vi "Goalie Normal.vi"(9 "balls":T1[](array[typedef]), 10 "Robot in":T3, 11 "IA State":T2={"our_robots"=[], "enemy_robots"=[], "balls"=[], "geometry"={"field_length"=0, "field_width"=0, "goal_width"=0, "goal_depth"=0, "center_circle_radius"=0, "defense_width"=0, "defense_depth"=0, "free_kick_from_defense_dist"=0, "penalty_spot_from_field_line_dist"=0, "penalty_line_from_spot_dist"=0, "half_moon_depth"=0, "half_moon_width"=0}, "IA Judge"={"stage"="", "command"="", "our_goalie_id"=0.0, "enemy_goalie_id"=0.0, "command enum"=enum."Halt", "Time"=enum."Azul"}, "Received Timestamp"=timestamp(0 s since 1904-01-01), "Events"={"Touch"=FALSE, "id touch"=0.0, "Ball out of \nVision"=FALSE, "Ball inside \nGoalie area"=FALSE, "Robot not responding"=FALSE, "Robots responding status"=[1.0, 1.0, 1.0, 1.0, 1.0, 1.0], "Enemy Ball \nPossession"=FALSE, "Id ini Possession"=0.0, "Ball Possesion"=FALSE, "Id Possesion"=0.0, "Ball at\nour goal side"=FALSE, "Ball at\ntouchline"=FALSE, "Ball at\nenemy goal side"=FALSE}}) -> (3 "Robot out":T3)   [LabVIEW 2017]
uses:
  Core/AI Robot.ctl
  Functions Enum.ctl
  AttackerStates.ctl
  Path Planning/RRT/PathDests.ctl
  Path Planning/RRT/PathDest.ctl
  Core/AI Input.ctl
  Core/AI Ball.ctl
  Core/Field Size.ctl
  Core/AI Judge.ctl
  Command Enum.ctl
  Util/Events/Events.ctl
  <vilib>/Analysis/_algsub.llb/Real Vector Norm.vi
  <vilib>/Analysis/NI_AALPro.lvlib
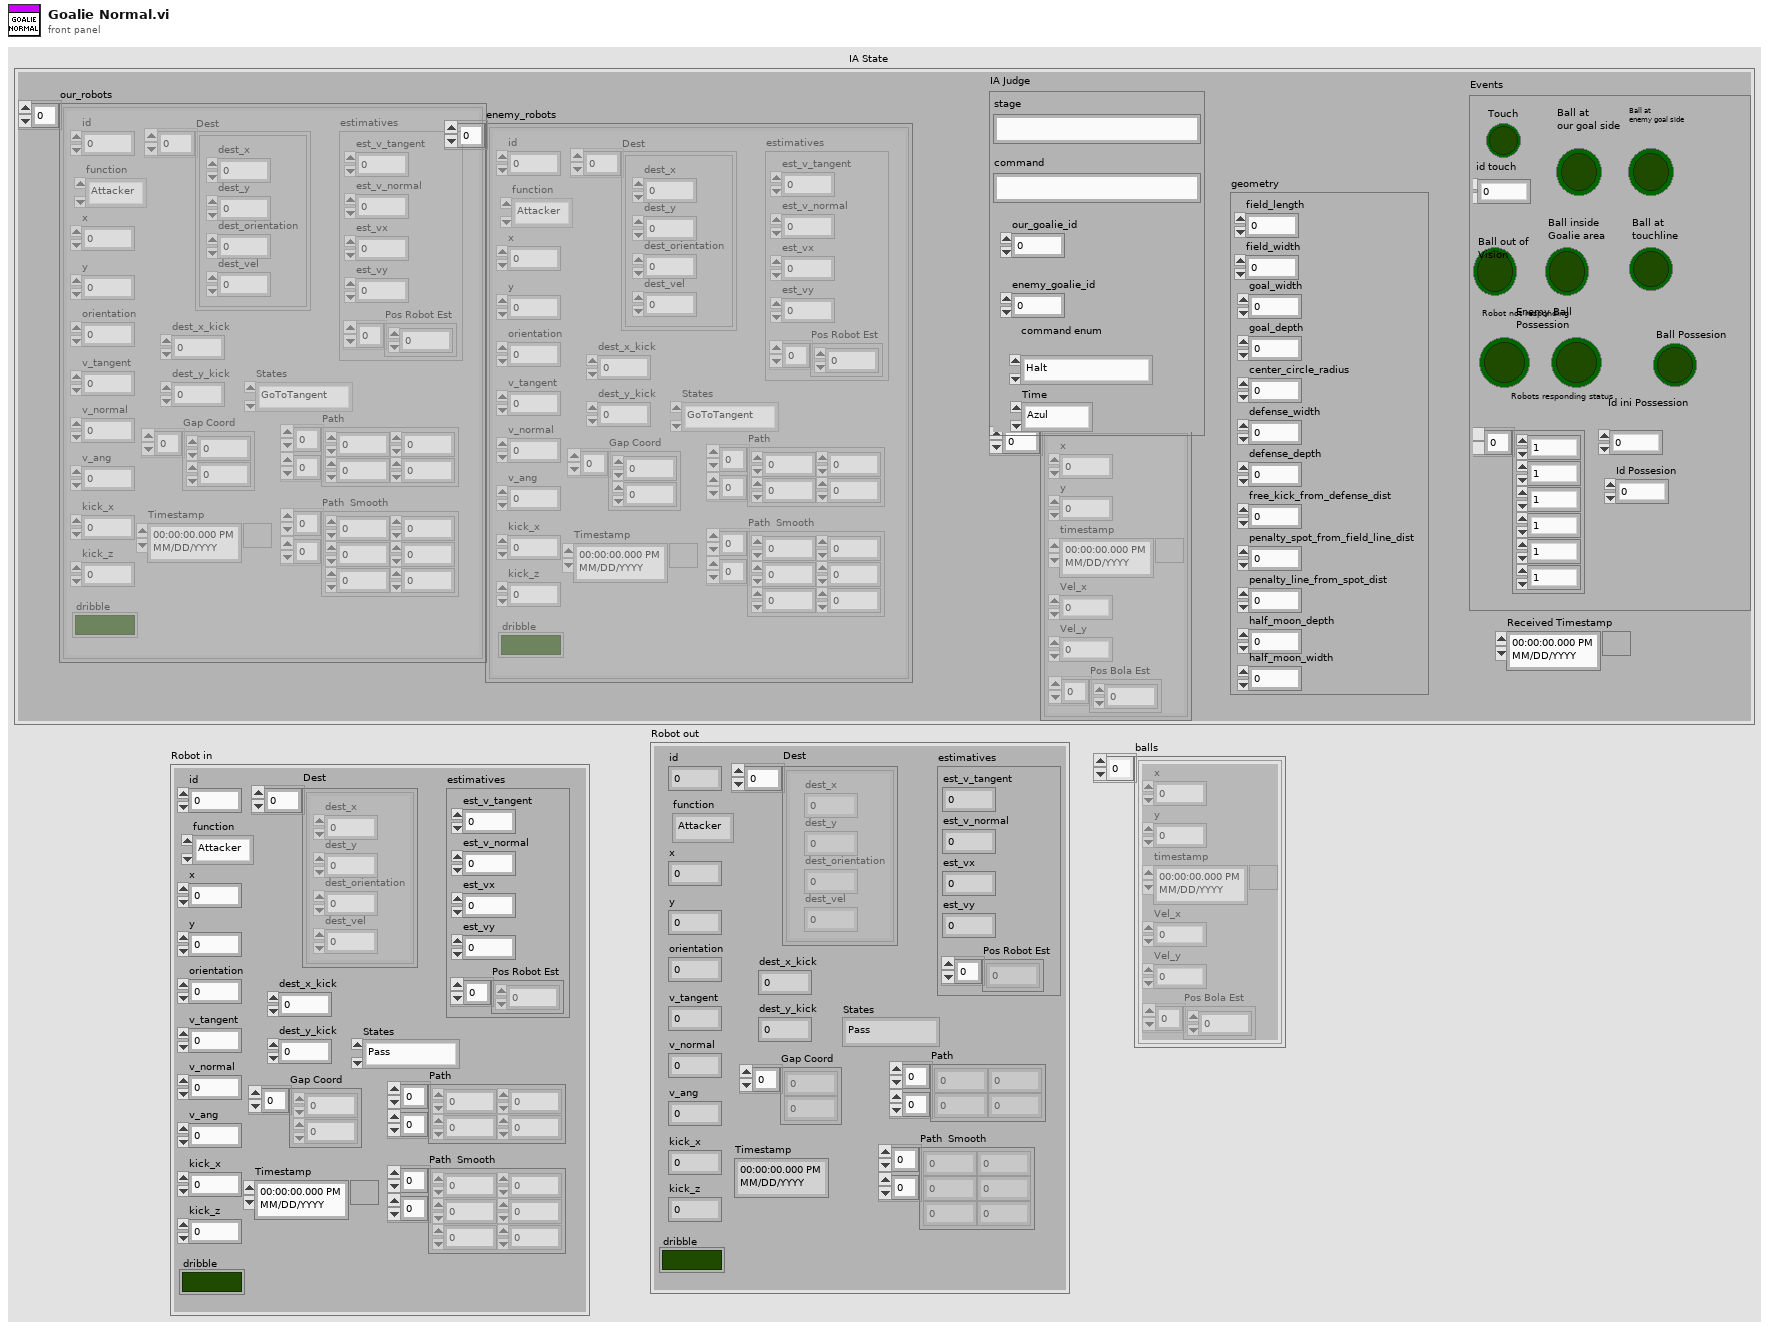
[diagram p1: front panel]
types:
  T1 = typedef "AI Ball.ctl" = cluster{"x":dbl, "y":dbl, "timestamp":timestamp, "Vel_x":dbl, "Vel_y":dbl, "Pos Bola Est":dbl[]}
  T2 = typedef "AI Input.ctl" = cluster{"our_robots":T3[], "enemy_robots":T3[], "balls":T1[], "geometry":T8, "IA Judge":T9, "Received Timestamp":timestamp, "Events":T11}
  T3 = typedef "AI Robot.ctl" = cluster{"id":u32, "function":T4, "x":dbl, "y":dbl, "orientation":dbl, "v_tangent":dbl, "v_normal":dbl, "v_ang":dbl, "kick_x":dbl, "kick_z":dbl, "dribble":bool, "Timestamp":timestamp, "estimatives":cluster{"est_v_tangent":dbl, "est_v_normal":dbl, "est_vx":dbl, "est_vy":dbl, "Pos Robot Est":dbl[]}, "dest_x_kick":dbl, "dest_y_kick":dbl, "Gap Coord":dbl[], "States":T5, "Path ":dbl[][], "Path  Smooth":dbl[][], "Dest":T6}
  T4 = typedef "Functions Enum.ctl" = enum16{"Attacker", "Goalie", "Defender", "Striker", "Goto 0", "Dummy", "Kicker", "ZigZag"}
  T5 = typedef "AttackerStates.ctl" = enum16{"Pass", "GoToTangent", "BallGetting", "GoToKick", "Rotate anti-clockwise", "Rotate Clockwise", ""}
  T6 = typedef "PathDests.ctl" = T7[]
  T7 = typedef "PathDest.ctl" = cluster{"dest_x":dbl, "dest_y":dbl, "dest_orientation":dbl, "dest_vel":dbl}
  T8 = typedef "Field Size.ctl" = cluster{"field_length":u32, "field_width":u32, "goal_width":u32, "goal_depth":u32, "center_circle_radius":u32, "defense_width":u32, "defense_depth":u32, "free_kick_from_defense_dist":u32, "penalty_spot_from_field_line_dist":u32, "penalty_line_from_spot_dist":u32, "half_moon_depth":u32, "half_moon_width":u32}
  T9 = typedef "AI Judge.ctl" = cluster{"stage":string, "command":string, "our_goalie_id":dbl, "enemy_goalie_id":dbl, "command enum":T10, "Time":enum16{"Azul", "Amarelo"}}
  T10 = typedef "Command Enum.ctl" = enum16{"Halt", "Stop", "Force Start", "PKA Normal Start", "Prepare Kickoff Ally", "PKE Normal Start", "Prepare Kickoff Enemy", "Prepare Penalty Ally", "PPA Normal Start", "Prepare Penalty Enemy", "PPE Normal Start", "Direct Free Enemy", "Direct Free Ally", "Indirect Free Enemy", "Indirect Free Ally", "Timeout Enemy", "Timeout Ally", "Goal Enemy", "Goal Ally", "Ball Placement Enemy", "Ball Placement Ally", "Normal Half Time", "Extra Time Break", "Extra Half Time", "None", "Post Game"}
  T11 = typedef "Events.ctl" = cluster{"Touch":bool, "id touch":dbl, "Ball out of \nVision":bool, "Ball inside \nGoalie area":bool, "Robot not responding":bool, "Robots responding status":dbl[], "Enemy Ball \nPossession":bool, "Id ini Possession":dbl, "Ball Possesion":bool, "Id Possesion":dbl, "Ball at\nour goal side":bool, "Ball at\ntouchline":bool, "Ball at\nenemy goal side":bool}
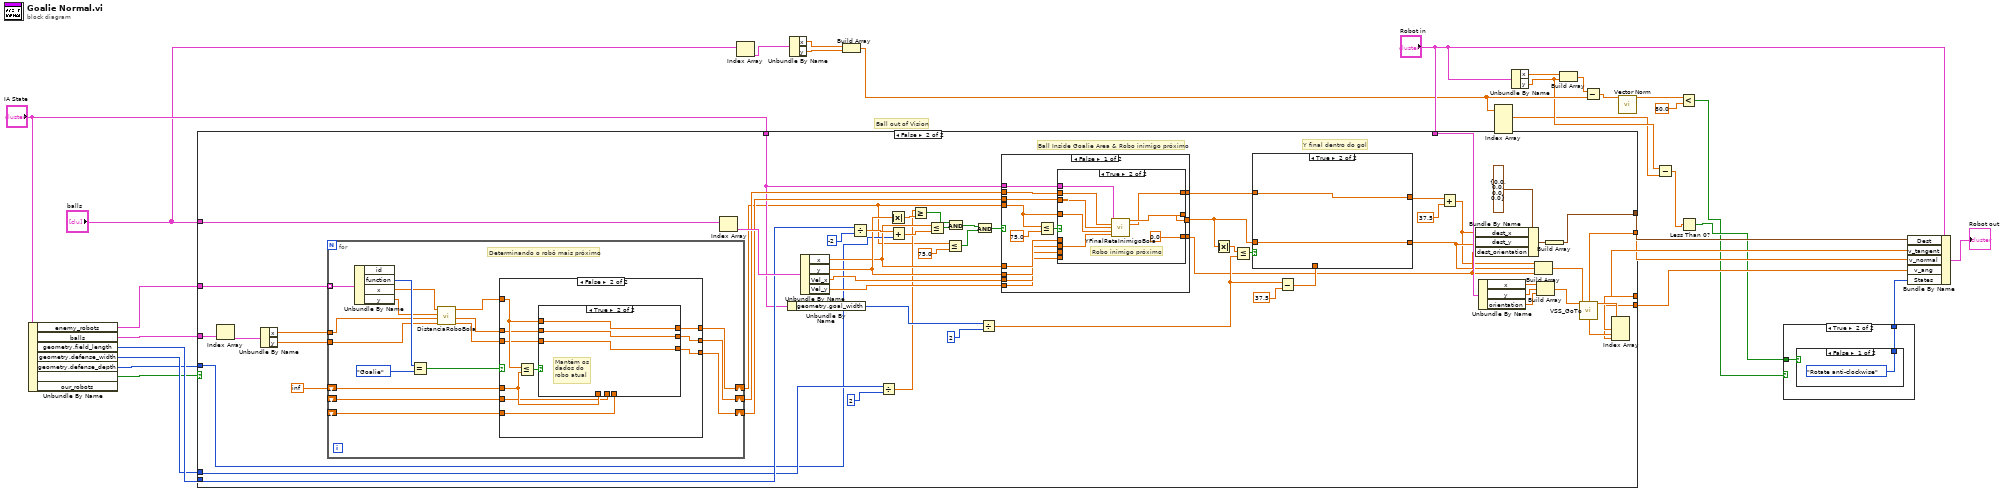
[diagram p0: block diagram]
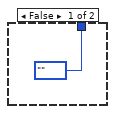
[diagram p2: hidden frame]
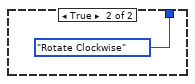
[diagram p3: hidden frame]
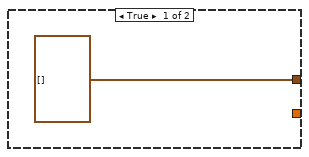
[diagram p4: hidden frame]
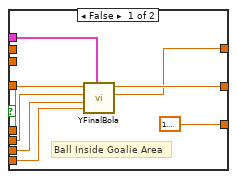
[diagram p5: hidden frame]
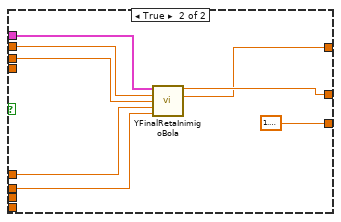
[diagram p6: hidden frame]
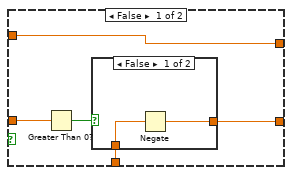
[diagram p7: hidden frame]
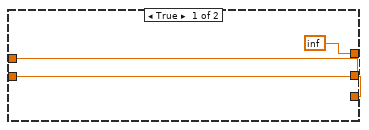
[diagram p9: hidden frame]
diagram:
  # "Ball out of Vision"
  n1 = Unbundle By Name("IA State") -> ("enemy_robots"=w26:T3[], "balls"=w27:T1[], "geometry.field_length"=w22:u32, "geometry.defense_width"=w20:u32, "geometry.defense_depth"=w19:u32, "Events.Ball out of \nVision"=w18:bool)  [unwired: 1 out]
  n2 = case shown="False" w18 {
    tunnel: [T7[] [] w88] -> w28
    tunnel: w27 -> [_ w84]
    tunnel: w26 -> [_ w83]
    tunnel: "balls" -> [_ w79]
    tunnel: "Robot in" -> [_ w71]
    tunnel: [_ w63] -> w25
    tunnel: [_ w62] -> w24
    tunnel: [_ w61] -> w23
    tunnel: w22 -> [_ w56]
    tunnel: "IA State" -> [_ w46]
    tunnel: w20 -> [_ w42]
    tunnel: w19 -> [_ w40]
    frame True {
    }
    frame False {
      # "Y final dentro do gol"
      # "Ball Inside Goalie Area & Robo inimigo próximo"
      n3 = Index Array(array=w84) -> (element=w85:T1)  [unwired: 1 in]
      n4 = Unbundle By Name(w85) -> ("x"=w82:dbl, "y"=w81:dbl)
      n5 = for {
        tunnel: w83 -> [w152] mode=indexing
        tunnel: w82 -> [w146]
        tunnel: w81 -> [w145]
        shift-right: [w139] -> w36
        shift-left: inf -> [w141]
        shift-right: [w137] -> w47
        shift-left: _ -> [w140]
        shift-right: [w136] -> w48
        shift-left: _ -> [w138]
        # "Determinando o robô mais próximo"
        n6 = Unbundle By Name(w152) -> ("function"=w150:T4, "x"=w148:dbl, "y"=w147:dbl)  [unwired: 1 out]
        n7 = Equal?(x=w150, y=Functions_Enum."Goalie") -> (x = y?=w149:bool)
        n8 = call "DistanciaRoboBola.vi"("Y bola"=w145, "X bola"=w146, "Y robo"=w147, "X robo"=w148) -> ("Y robo"=w142:dbl, "X robo"=w143:dbl, "Distância"=w144:dbl)  [unwired: 5 in]
        n9 = case shown="False" w149 {
          tunnel: w144 -> [_ w163]
          tunnel: w143 -> [w154 w162]
          tunnel: w142 -> [w153 w161]
          tunnel: w141 -> [_ w160]
          tunnel: w140 -> [_ w159]
          tunnel: [inf w165] -> w139
          tunnel: w138 -> [_ w156]
          tunnel: [w154 w158] -> w137
          tunnel: [w153 w157] -> w136
          frame True {
          }
          frame False {
            n10 = Less Or Equal?(x=w163, y=w160) -> (x <= y?=w164:bool)
            n11 = case shown="True" w164 {
              tunnel: [w167 w170] -> w158
              tunnel: [w168 w171] -> w165
              tunnel: w163 -> [_ w171]
              tunnel: w162 -> [_ w170]
              tunnel: w161 -> [_ w169]
              tunnel: w160 -> [w168 _]
              tunnel: w159 -> [w167 _]
              tunnel: w156 -> [w166 _]
              tunnel: [w166 w169] -> w157
              frame False {
                # "Mantém os\ndados do\nrobo anterior"
              }
              frame True {
                # "Mantém os\ndados do\nrobo atual"
              }
            }
          }
        }
      }
      n12 = Index Array(array=w79) -> (element=w78:T1)  [unwired: 1 in]
      n13 = Unbundle By Name(w46) -> ("geometry.goal_width"=w59:u32)
      n14 = Unbundle By Name(w78) -> ("x"=w49:dbl, "y"=w50:dbl, "Vel_x"=w51:dbl, "Vel_y"=w52:dbl)
      n15 = Divide(x=w56, y=-2) -> (x/y=w55:dbl)
      n16 = Divide(x=w42, y=2) -> (x/y=w41:dbl)
      n17 = Absolute Value(x=w50) -> (abs(x)=w60:dbl)
      n18 = Add(x=w55, y=w40) -> (x+y=w54:dbl)
      n19 = Greater Or Equal?(x=w41, y=w60) -> (x >= y?=w58:bool)
      n20 = Less Or Equal?(x=w49, y=w54) -> (x <= y?=w53:bool)
      n21 = Less Or Equal?(x=w36, y=75.0) -> (x <= y?=w35:bool)
      n22 = And(x=w58, y=w53) -> (x .and. y?=w38:bool)
      n23 = And(x=w38, y=w35) -> (x .and. y?=w39:bool)
      n24 = Divide(x=w59, y=2) -> (x/y=w73:dbl)
      n25 = case shown="False" w39 {
        tunnel: w52 -> [w91 _]
        tunnel: w51 -> [w92 _]
        tunnel: w50 -> [w93 w121]
        tunnel: w49 -> [w94 w122]
        tunnel: w36 -> [w95 _]
        tunnel: w48 -> [w96 w123]
        tunnel: w47 -> [w97 w124]
        tunnel: w46 -> [w98 w125]
        tunnel: [w99 w119] -> w45
        tunnel: [w100 w120] -> w44
        tunnel: [w89 1.5707963267948966] -> w34
        frame False {
          n26 = Less Or Equal?(x=w95, y=75.0) -> (x <= y?=w90:bool)
          n27 = case shown="True" w90 {
            tunnel: w98 -> [w103 w116]
            tunnel: w97 -> [_ w115]
            tunnel: w96 -> [_ w114]
            tunnel: w94 -> [w109 _]
            tunnel: w93 -> [w108 w113]
            tunnel: [w105 w117] -> w100
            tunnel: w92 -> [w107 _]
            tunnel: w91 -> [w106 _]
            tunnel: [w104 w112] -> w99
            tunnel: w95 -> [_ w111]
            tunnel: [1.5707963267948966 0.0] -> w89
            frame False {
              # "Ball Inside Goalie Area"
              n28 = call "YFinalBola.vi"("IA State"=w103, "Vy bola"=w106, "Vx bola"=w107, "Y bola"=w108, "X bola"=w109) -> ("X goleiro"=w104:dbl, "Y final da bola"=w105:dbl)  [unwired: 5 in]
            }
            frame True {
              # "Robo inimigo próximo"
              n29 = call "YFinalRetaInimigoBola.vi"("IA State"=w116, "X robo"=w115, "Y robo"=w114, "X bola"=w111, "Y bola"=w113) -> ("Y final da bola"=w117:dbl, "X goleiro"=w112:dbl)  [unwired: 9 in]
            }
          }
        }
        frame True {
          n30 = call "YFinalRetaInimigoBola.vi"("IA State"=w125, "X robo"=w124, "Y robo"=w123, "X bola"=w122, "Y bola"=w121) -> ("Y final da bola"=w120:dbl, "X goleiro"=w119:dbl)  [unwired: 9 in]
        }
      }
      n31 = Absolute Value(x=w44) -> (abs(x)=w77:dbl)
      n32 = Less Or Equal?(x=w77, y=w73) -> (x <= y?=w75:bool)
      n33 = Subtract(x=w73, y=37.5) -> (x-y=w72:dbl)
      n34 = case shown="True" w75 {
        tunnel: w44 -> [w130 w135]
        tunnel: [w127 w135] -> w66
        tunnel: [w126 w134] -> w33
        tunnel: w45 -> [w126 w134]
        tunnel: w72 -> [w128 _]
        frame False {
          n35 = Greater Than 0?(x=w130) -> (x > 0?=w129:bool)
          n36 = case shown="False" w129 {
            tunnel: [w131 w133] -> w127
            tunnel: w128 -> [w132 w133]
            frame False {
              n37 = Negate(x=w132) -> (-x=w131:dbl)
            }
            frame True {
            }
          }
        }
        frame True {
        }
      }
      n38 = Add(x=w33, y=37.5) -> (x+y=w31:dbl)
      n39 = Bundle By Name(cluster=T7 {"dest_x"=0.0, "dest_y"=0.0, "dest_orientation"=0.0, "dest_vel"=0.0} ("element"), "dest_x"=w31, "dest_y"=w66, "dest_orientation"=w34) -> (w87:T7)
      n40 = Unbundle By Name(w71) -> ("x"=w67:dbl, "y"=w70:dbl, "orientation"=w69:dbl)
      n41 = Build Array(w31, w66, w34) -> (w65:dbl[])
      n42 = Build Array(w67, w70, w69) -> (w68:dbl[])
      n43 = Build Array(w87) -> (w88:T7[])
      n44 = call "VSS_GoTo.vi"("SetPoint"=w65, "Position"=w68) -> ("Output Vel"=w64:dbl[])  [unwired: 9 in]
      n45 = Index Array(array=w64) -> (element #1=w63:dbl, element #2=w62:dbl, element #3=w61:dbl)  [unwired: 3 in]
    }
  }
  n46 = Index Array(array="balls") -> (element=w14:T1)  [unwired: 1 in]
  n47 = Unbundle By Name(w14) -> ("x"=w13:dbl, "y"=w12:dbl)
  n48 = Build Array(w13, w12) -> (w6:dbl[])
  n49 = Index Array(array=w6) -> (element #1=w3:dbl)  [unwired: 4 in, 3 out]
  n50 = Unbundle By Name("Robot in") -> ("x"=w16:dbl, "y"=w5:dbl)
  n51 = Build Array(w16, w5) -> (w11:dbl[])
  n52 = Subtract(x=w11, y=w6) -> (x-y=w9:dbl[])
  n53 = call-poly <vilib>:"Vector Norm.vi"("Input Vector"=w9) -> ("norm"=w8:dbl)  [unwired: 9 in, 1 out]
  n54 = Subtract(x=w5, y=w3) -> (x-y=w4:dbl)
  n55 = Less?(x=w8, y=80.0) -> (x < y?=w1:bool)
  n56 = Less Than 0?(x=w4) -> (x < 0?=w2:bool)
  n57 = case shown="True" w1 {
    tunnel: [AttackerStates."" ("States") w174] -> w7
    tunnel: w2 -> [_ w173]
    frame False {
    }
    frame True {
      n58 = case shown="False" w173 {
        tunnel: [AttackerStates."Rotate anti-clockwise" ("States") AttackerStates."Rotate Clockwise" ("States")] -> w174
        frame False {
        }
        frame True {
        }
      }
    }
  }
  n59 = Bundle By Name(cluster="Robot in", "Dest"=w28, "v_tangent"=w25, "v_normal"=w24, "v_ang"=w23, "States"=w7) -> (→"Robot out":T3)
